vi "SNAKE_LADER.vi"() -> ()   [LabVIEW 2018]
panel:
  out "x":dbl
  out "y":dbl
  # "98"
  # "93"
  # "94"
  # "97"
  # "95"
  # "100"
  # "91"
  # "92"
  # "99"
  # "96"
  # "87"
  # "85"
  # "90"
  # "89"
  # "82"
  # "84"
  # "88"
  # "86"
  # "83"
  # "81"
  # "80"
  # "74"
  # "78"
  # "72"
  # "75"
  # "76"
  # "77"
  # "79"
  # "71"
  # "73"
  # "61"
  # "62"
  # "67"
  # "68"
  # "69"
  # "64"
  # "66"
  # "65"
  # "70"
  # "63"
  # "57"
  # "52"
  # "53"
  # "58"
  # "54"
  # "55"
  # "56"
  # "59"
  # "51"
  # "60"
  # "45"
  # "46"
  # "47"
  # "43"
  # "42"
  # "48"
  # "49"
  # "50"
  # "41"
  # "44"
  # "31"
  # "33"
  # "35"
  # "37"
  # "32"
  # "36"
  # "39"
  # "34"
  # "40"
  # "38"
  # "27"
  # "26"
  # "30"
  # "22"
  # "23"
  # "24"
  # "29"
  # "21"
  # "25"
  # "28"
  # "15"
  # "17"
  # "11"
  # "12"
  # "19"
  # "20"
  # "14"
  # "16"
  # "13"
  # "18"
  # "8"
  # "7"
  # "3"
  # "1"
  # "2"
  # "4"
  # "5"
  # "9"
  # "10"
  # "6"
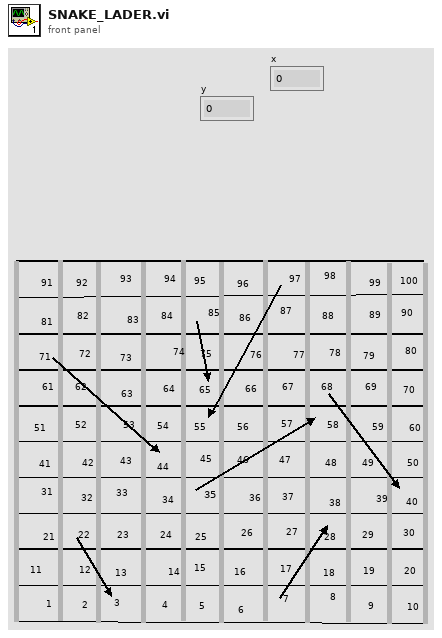
[diagram p1: front panel]
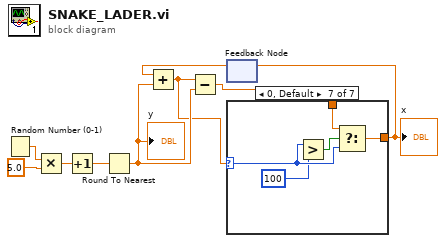
[diagram p0: block diagram]
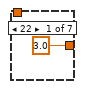
[diagram p2: hidden frame]
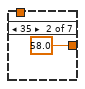
[diagram p3: hidden frame]
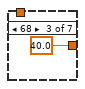
[diagram p4: hidden frame]
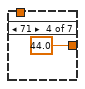
[diagram p5: hidden frame]
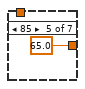
[diagram p6: hidden frame]
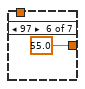
[diagram p7: hidden frame]
diagram:
  n1 = Random Number (0-1)() -> (number: 0 to 1=w9:dbl)
  n2 = Multiply(x=w9, y=5.0) -> (x*y=w7:dbl)
  n3 = Increment(x=w7) -> (x+1=w6:dbl)
  n4 = Round To Nearest(number=w6) -> (nearest integer value=w3:dbl)
  "y" <- w3
  n5 = feedback #1() -> (w5:dbl)  [unwired: 1 in]
  n6 = Add(x=w5, y=w3) -> (x+y=w2:dbl)
  n7 = Subtract(x=w2, y=w3) -> (x-y=w1:dbl)
  n8 = case shown="0, Default" w2 {
    selector: w2 -> [_ _ _ _ _ _ w17]
    tunnel: [3.0 ("f") 58.0 ("f") 40.0 ("f") 44.0 ("f") 65.0 ("f") 55.0 ("f") w19] -> w4
    tunnel: w1 -> [_ _ _ _ _ _ w18]
    frame 22 {
    }
    frame 35 {
    }
    frame 68 {
    }
    frame 71 {
    }
    frame 85 {
    }
    frame 97 {
    }
    frame 0, Default {
      n9 = Greater?(x=w17, y=100 ("x")) -> (0:w20:bool)
      n10 = Select(t=w18, s=w20, f=w17) -> (s? t:f=w19:dbl)
    }
  }
  "x" <- w4
  n11 = feedback-in #1(w4) -> ()
